vi "PV HLT5xx Set Pressure Data.vi"(1 "Value in":dbl=1e-09 min=1e-09 max=1000.0 step=1e-09 format="%.2e") -> (0 "Output":string)   [LabVIEW 2016, in "Pfeiffer Vacuum.lvlib"]
uses:
  Pfeiffer Vacuum.lvlib
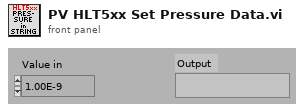
[diagram p1: front panel]
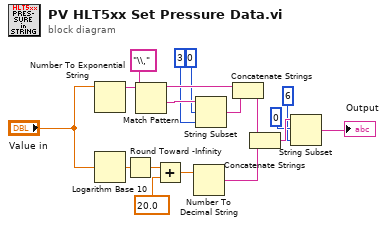
[diagram p0: block diagram]
diagram:
  n1 = Number To Exponential String(number="Value in") -> (E-format string=w12:string)  [unwired: 3 in]
  n2 = Logarithm Base 10(1:"Value in") -> (0:w16:dbl)
  n3 = Round Toward -Infinity(1:w16) -> (0:w15:dbl)
  n4 = Match Pattern(string=w12, regular expression="\\,") -> (before substring=w13:string, after substring=w11:string)  [unwired: 1 in, 2 out]
  n5 = Add(x=w15, y=20.0) -> (x+y=w7:dbl)
  n6 = Number To Decimal String(number=w7) -> (decimal integer string=w4:string)  [unwired: 1 in]
  n7 = String Subset(string=w11, offset (0)=0 ("Offset (0)"), length (rest)=3 ("Länge")) -> (substring=w8:string)
  n8 = Concatenate Strings(w13, w8) -> (w5:string)
  n9 = Concatenate Strings(w5, w4) -> (w3:string)
  n10 = String Subset(string=w3, offset (0)=0 ("Offset (0)"), length (rest)=6 ("Länge")) -> (substring=→"Output":string)
